vi "Write Server Actor.vi"(8 "error in (no error)":errorcluster, 10 "Server Actor":string, 11 "DIMDemoClient in":refnum<class "DIMDemoClient.lvclass">) -> (0 "error out":errorcluster, 3 "DIMDemoClient out":refnum<class "DIMDemoClient.lvclass">)   [LabVIEW 2012, in "DimActorDemo.lvlib" / "DIMDemoClient.lvclass"]
doc: "Write server actor."
uses:
  DIMDemoClient.lvclass
  DIMDemoClient.lvclass/DIMDemoClient.ctl
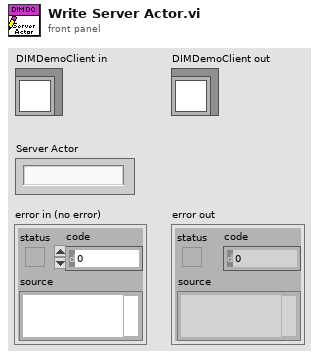
[diagram p1: front panel]
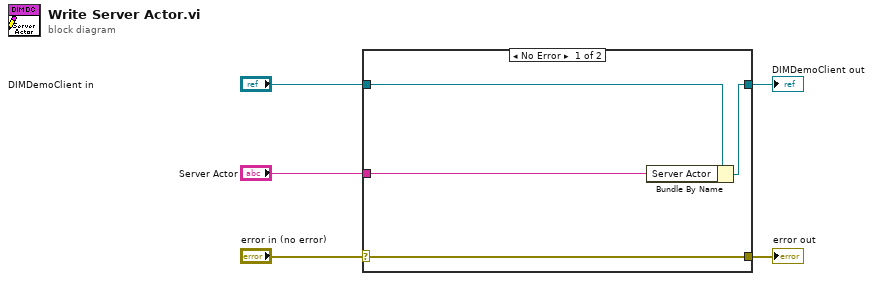
[diagram p0: block diagram]
diagram:
  n1 = case shown="No Error" "error in (no error)" {
    selector: "error in (no error)" -> [w9 w10]
    tunnel: [w9 w10] -> w4
    tunnel: [w7 w11] -> w2
    tunnel: "DIMDemoClient in" -> [w8 w11]
    tunnel: "Server Actor" -> [w6 _]
    frame No Error {
      n2 = Bundle By Name(cluster=w8, "Server Actor"=w6) -> (w7:refnum<class "DIMDemoClient.lvclass">)
    }
    frame Error {
    }
  }
  "error out" <- w4
  "DIMDemoClient out" <- w2
